vi "Analysis.FG, Data Value Items.vi"(6 "ResultID":i32, 7 "Action":T1=enum."Add Value", 8 "UL":string, 9 "LL":string, 10 "Value":string, 11 "Name":string) -> (0 "error out":errorcluster, 1 "2DVals Out":string[][](array[string]), 2 "Name/1DVals Out":string[](array[string]), 3 "Limits":variant, 4 "1DVals Num":dbl[](array[numeric]))   [LabVIEW 2024]
uses:
  Analysis.Data Value Items Action.ctl
  Analysis.Measurement Limit Info.ctl
  <vilib>/KATE/Files/File Utils.lvlib
  <vilib>/KATE/Strings/String Utils.lvlib
panel:
  # "Init\n  Clear Data\n\nAdd Value:\n  Inputs:\n    ResultID\n    Name\n    Val\n    LL\n    UL\n  Outputs:\n    None\n\nGet Meas Num Values \n  Used for Graphs\n  Inputs:\n    Name\n  Outputs:\n    1D Num Values\n       Indices align with TestResultID\n\nGet Meas Num Values Only \n  Used for Stats\n  Inputs:\n    Name\n  Outputs:\n    1D Num Values\n       Array of numeric data only\n\nDump All:\n   Outputs:\n     Var Limits\n     1D Names\n     2D Values"
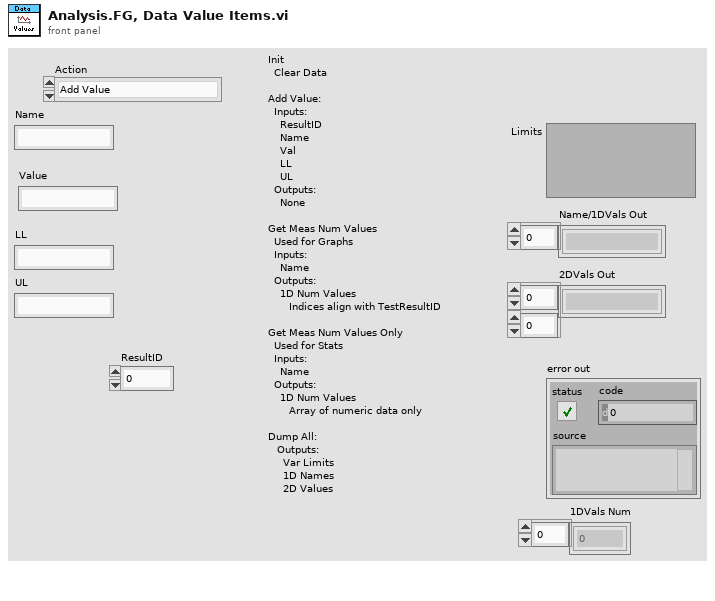
[diagram p1: front panel]
types:
  T1 = typedef "Analysis.Data Value Items Action.ctl" = enum16{"Init", "Add Value", "Get MeasVals", "Get Lists", "Get RsltVals", "Dump All", "Dump Vals to File", "Get Rslt Meas Val", "Dump Lists to File", "Load Values from File", "Load Lists From File", "Get MeasVals Num Only", "TrimDataTable"}
  T2 = typedef "Analysis.Measurement Limit Info.ctl" = cluster{"Name":string, "Numeric":bool, "LL":dbl, "LL_En":bool, "UL":dbl, "UL_En":bool, "Units":string}
  T3 = enum16{"open", "replace", "create", "open or create", "replace or create", "replace or create with confirmation"}
  T4 = cluster{"Names":string[], "MeasDims_Out":variant}
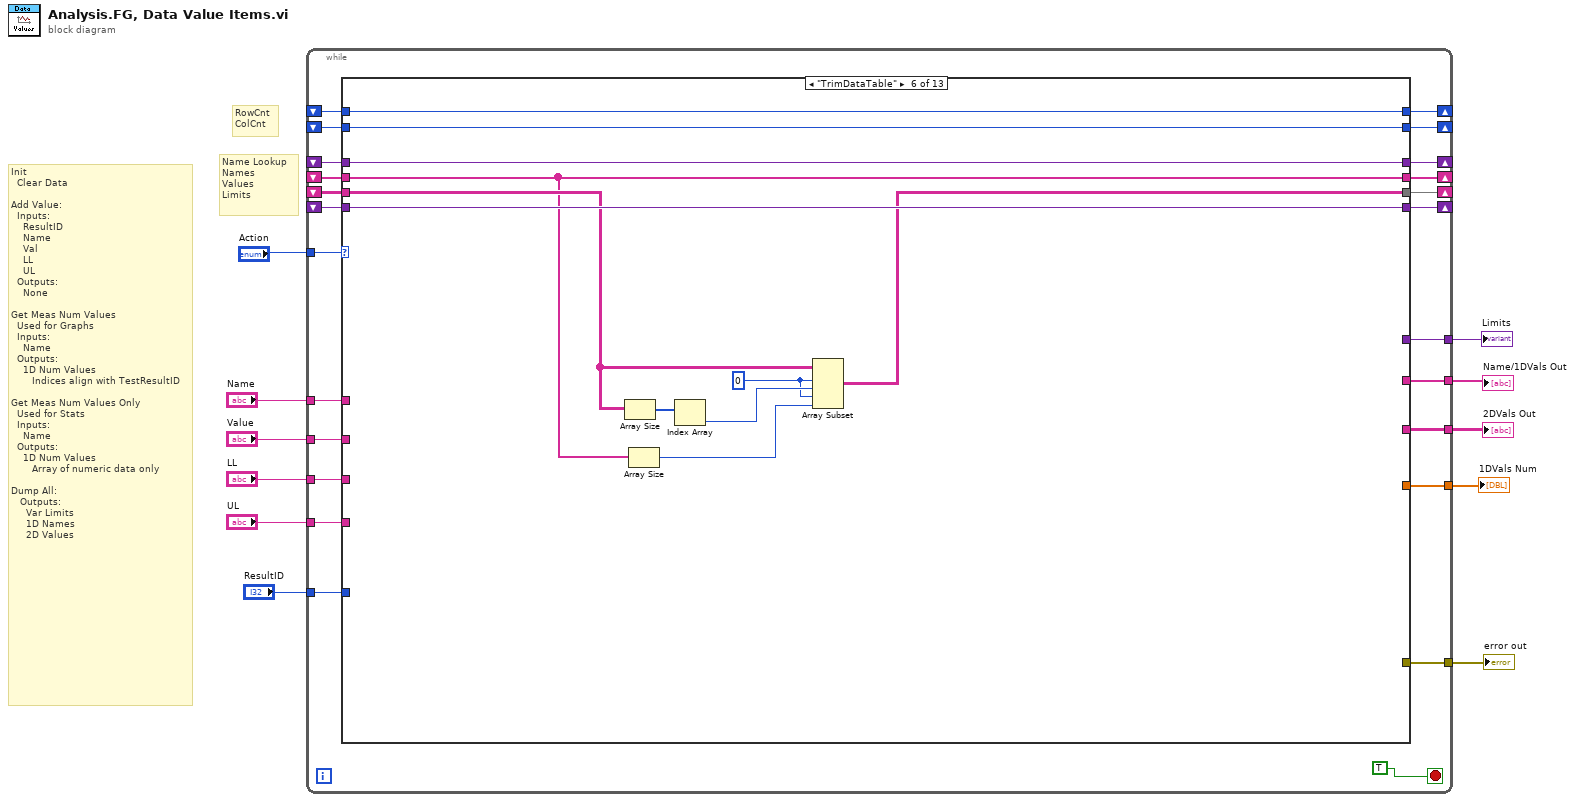
[diagram p0: block diagram]
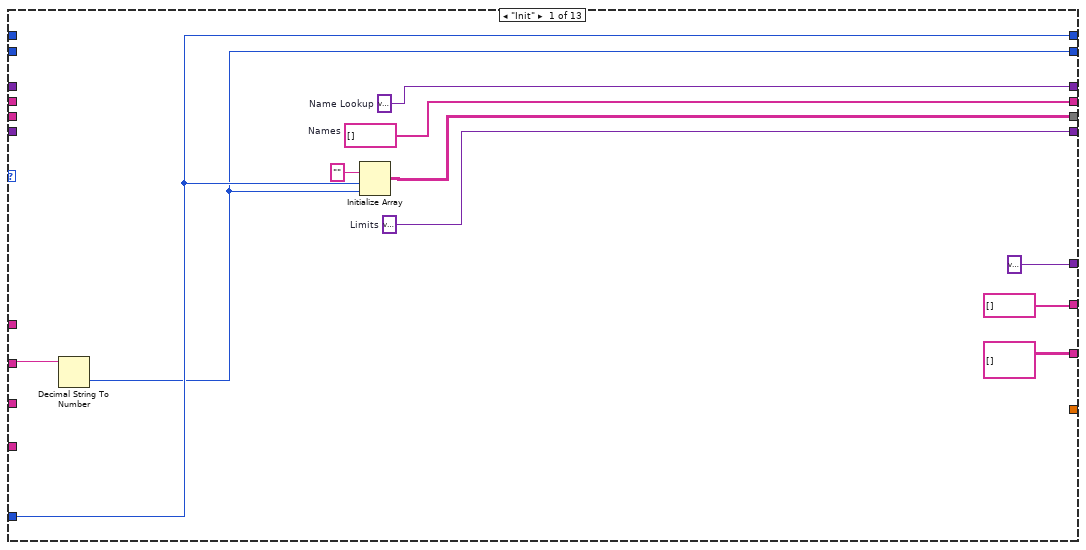
[diagram p2: hidden frame]
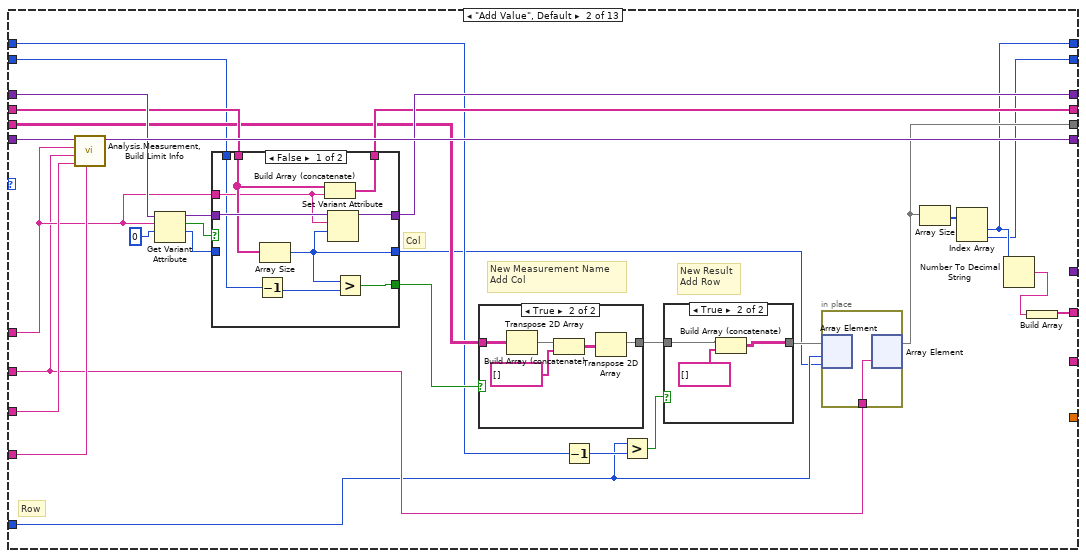
[diagram p3: hidden frame]
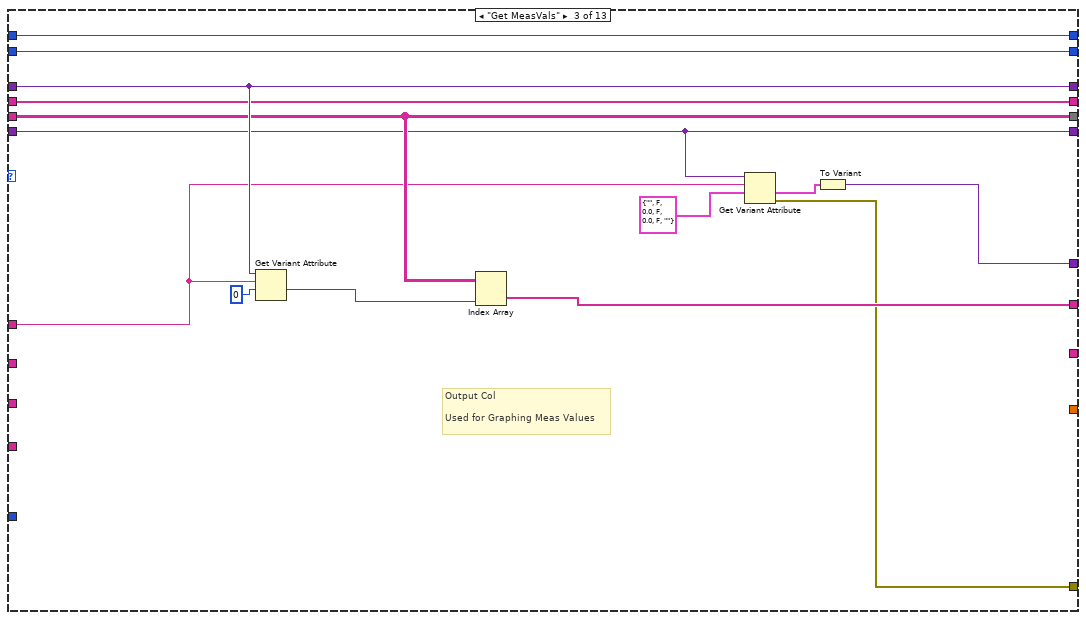
[diagram p7: hidden frame]
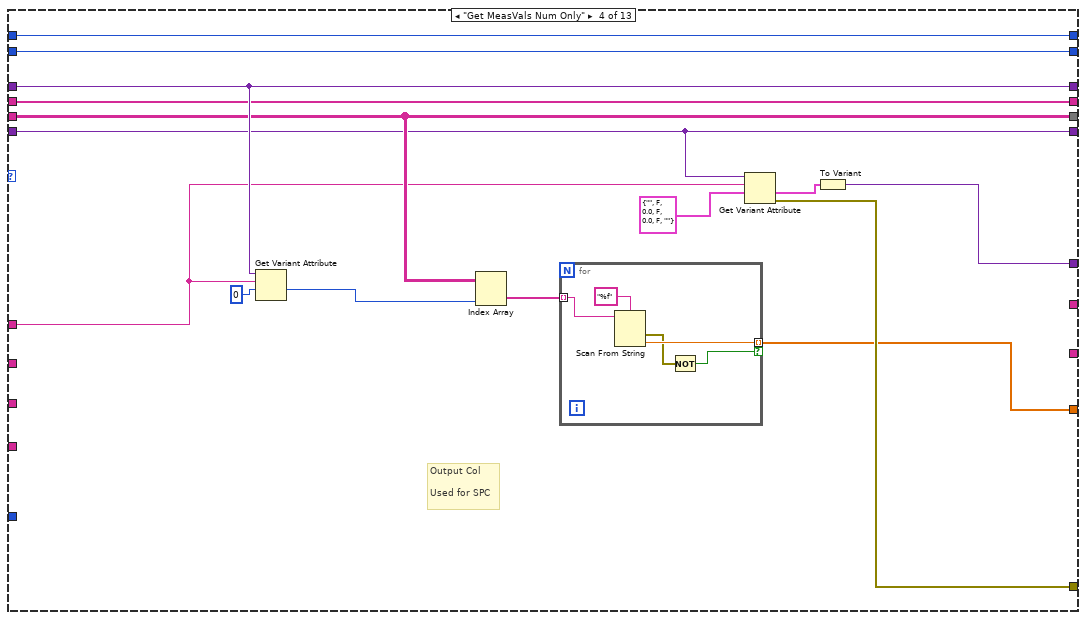
[diagram p8: hidden frame]
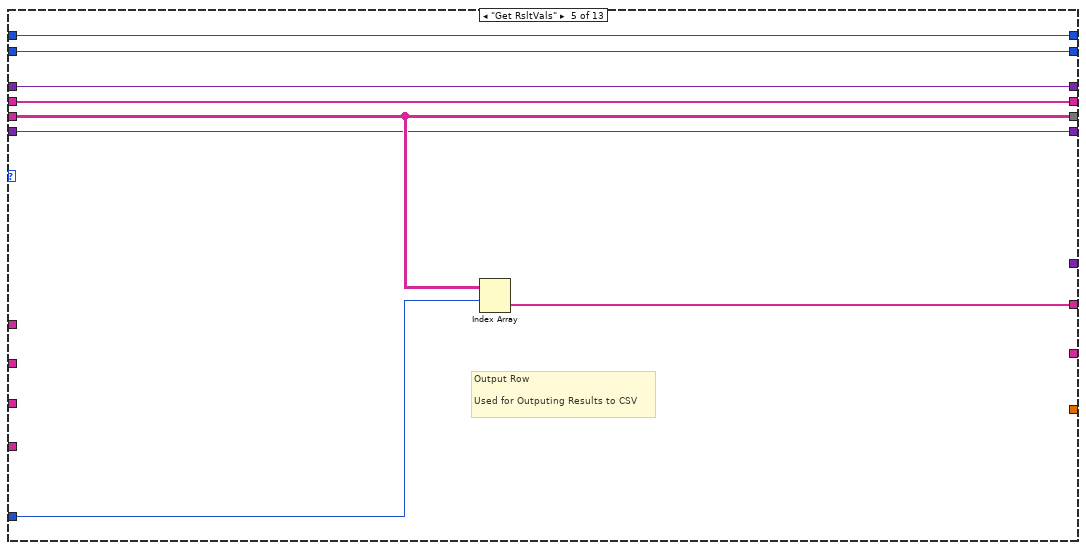
[diagram p9: hidden frame]
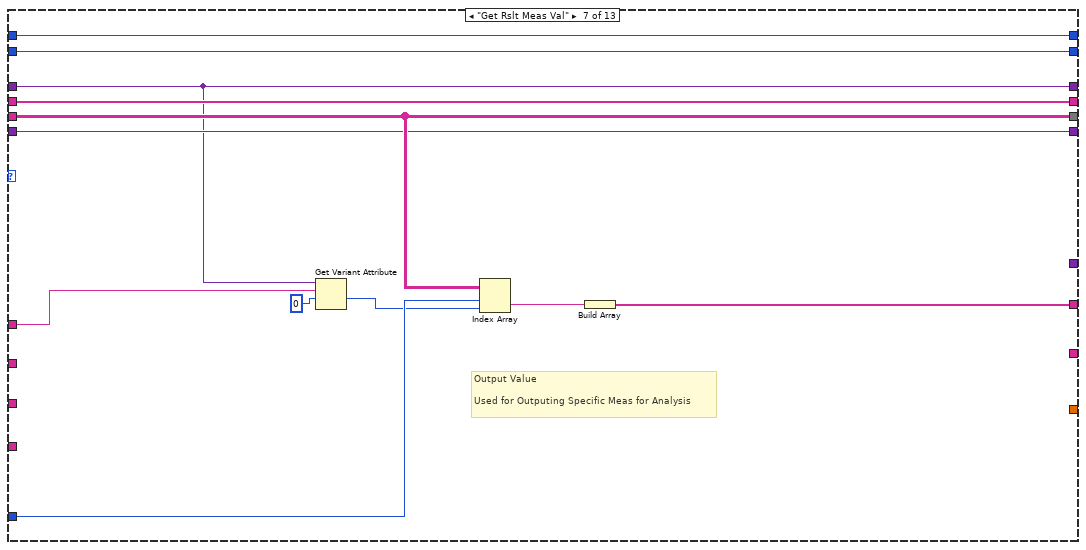
[diagram p10: hidden frame]
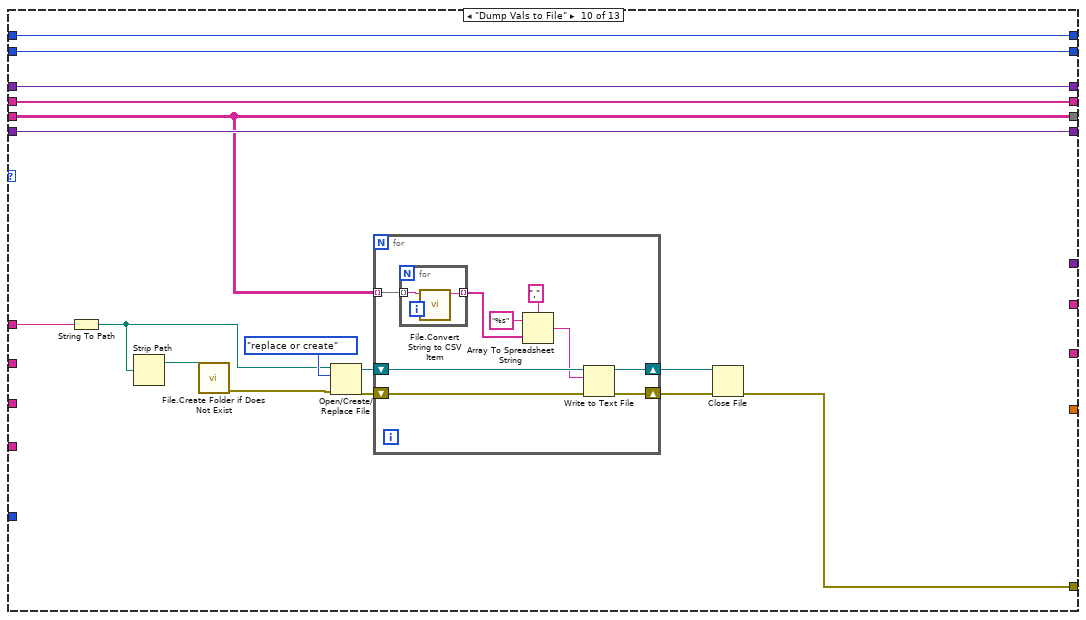
[diagram p13: hidden frame]
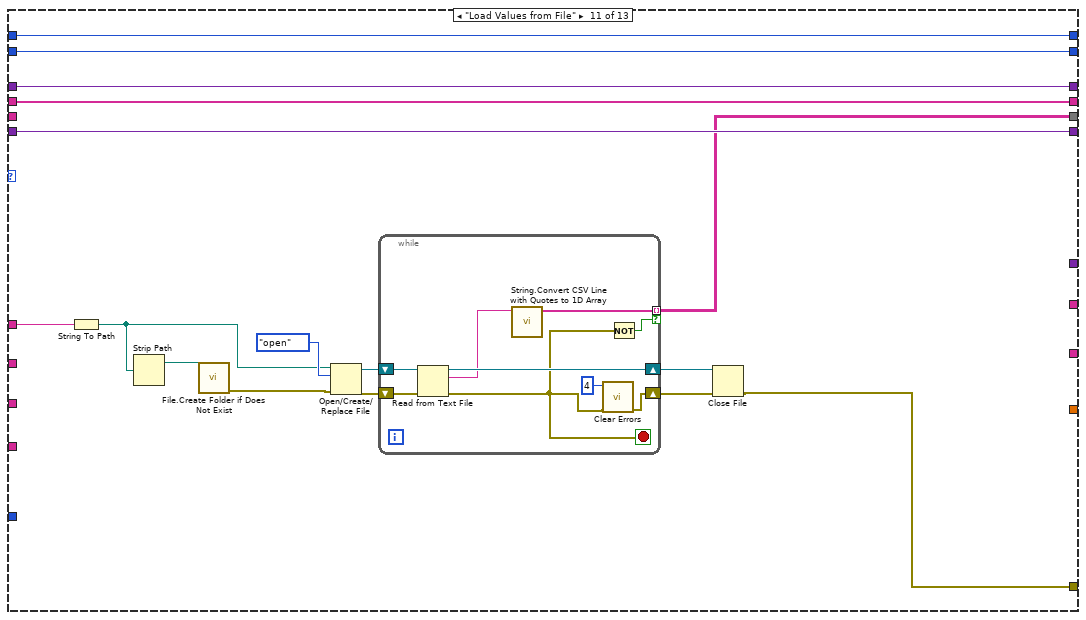
[diagram p14: hidden frame]
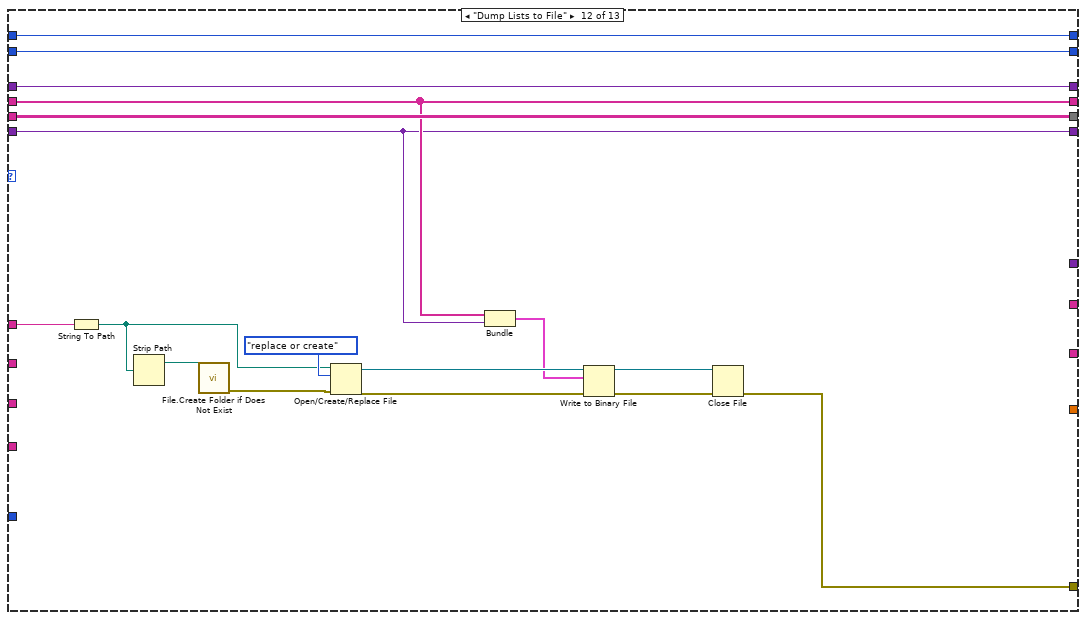
[diagram p15: hidden frame]
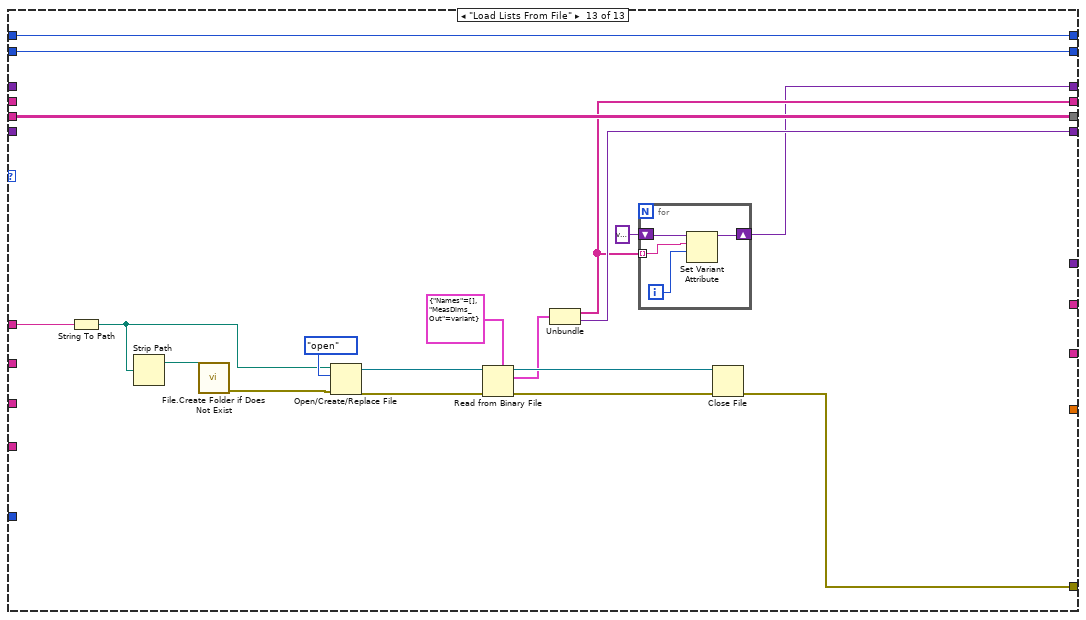
[diagram p16: hidden frame]
diagram:
  # "RowCnt\nColCnt"
  # "Init\n  Clear Data\n\nAdd Value:\n  Inputs:\n    ResultID\n    Name\n    Val\n    LL\n    UL\n  Outputs:\n    None\n\nGet Meas Num Values \n  Used for Graphs\n  Inputs:\n    Name\n  Outputs:\n    1D Num Values\n       Indices align with TestResultID\n\nGet Meas Num Values Only \n  Used for Stats\n  Inputs:\n    Name\n  Outputs:\n    1D Num Values\n       Array of numeric data only\n\nDump All:\n   Outputs:\n     Var Limits\n     1D Names\n     2D Values"
  # "Name Lookup\nNames\nValues\nLimits"
  n1 = while {
    tunnel: "Action" -> [w35]
    shift-right: [w29] -> _
    shift-left: _ -> [w34]
    shift-right: [w28] -> _
    shift-left: _ -> [w33]
    shift-right: [w27] -> _
    shift-left: _ -> [w32]
    shift-right: [w30] -> _
    shift-left: _ -> [w31]
    tunnel: "ResultID" -> [w26]
    tunnel: "Name" -> [w25]
    tunnel: "Value" -> [w24]
    tunnel: "LL" -> [w23]
    tunnel: "UL" -> [w22]
    tunnel: [w21] -> w5
    tunnel: [w20] -> w4
    tunnel: [w19] -> w3
    tunnel: [w17] -> w2
    tunnel: [w16] -> w1
    shift-right: [w15] -> _
    shift-left: _ -> [w13]
    shift-right: [w14] -> _
    shift-left: _ -> [w12]
    stop <- TRUE stop-if-true
    n2 = case shown="\"TrimDataTable\"" w35 {
      tunnel: w34 -> [_ w76 w107 w123 w139 w151 w163 w167 w175 w191 w218 w233 _]
      tunnel: [w37 w49 w111 w126 w140 w142 w164 w170 w173 w180 w207 w235 w255] -> w28
      tunnel: [w46 w66 w109 w124 w138 w144 w162 w168 w174 w190 w217 w234 w250] -> w27
      tunnel: w33 -> [_ w60 w111 w126 w140 w148 w164 w170 w173 w180 _ w235 w255]
      tunnel: w32 -> [_ w67 w109 w124 w138 w144 w162 w168 w174 w190 w217 w234 _]
      tunnel: w31 -> [_ w70 w112 w127 w141 w152 w159 w169 w176 w192 w219 w245 _]
      tunnel: [w45 w69 w112 w127 w141 w152 w159 w169 w176 w192 w219 w245 w248] -> w30
      tunnel: [w44 w73 w107 w123 w139 w151 w163 w167 w175 w191 w218 w233 w252] -> w29
      tunnel: w26 -> [w40 w51 _ _ w137 _ w161 _ _ _ _ _ _]
      tunnel: w25 -> [_ w68 w105 w121 _ _ w158 _ _ w189 w216 w244 w264]
      tunnel: w24 -> [w36 w52 _ _ _ _ _ _ _ _ _ _ _]
      tunnel: w23 -> [_ w75 _ _ _ _ _ _ _ _ _ _ _]
      tunnel: w22 -> [_ w74 _ _ _ _ _ _ _ _ _ _ _]
      tunnel: [variant ("Var Out") _ w102 w118 _ _ _ w167 w175 _ _ _ _] -> w21
      tunnel: [string[] [] ("1D Str Out") w57 w108 _ w136 _ w155 w168 w174 _ _ _ _] -> w20
      tunnel: [string[][] [] ("2D Str Out") _ _ _ _ _ _ _ w173 _ _ _ _] -> w19
      tunnel: [_ _ w104 w120 _ _ _ _ _ w179 w206 w231 w251] -> w17
      tunnel: [_ _ _ w116 _ _ _ _ _ _ _ _ _] -> w16
      tunnel: [w40 w48 w101 w115 w135 w150 w154 w166 w172 w178 w205 w230 w247] -> w15
      tunnel: [w39 w47 w100 w114 w134 w149 w153 w165 w171 w177 w204 w229 w246] -> w14
      tunnel: w13 -> [_ w55 w101 w115 w135 w150 w154 w166 w172 w178 w205 w230 w247]
      tunnel: w12 -> [_ w54 w100 w114 w134 w149 w153 w165 w171 w177 w204 w229 w246]
      frame "Init" {
        w45 = variant  # Name Lookup
        w44 = variant  # Limits
        w46 = string[] []  # Names
        n3 = Decimal String To Number(string=w36) -> (number=w39:i32)  [unwired: 2 in, 1 out]
        n4 = Initialize Array("", w40, w39) -> (w37:string[][])
      }
      frame "Add Value", Default {
        # "New Measurement Name\nAdd Col"
        # "New Result\nAdd Row"
        # "Col"
        # "Row"
        n5 = call "Analysis.Measurement, Build Limit Info.vi"("UL"=w74, "LL"=w75, "Value"=w52, "Name"=w68, "MeasDims_In"=w76) -> ("MeasDims_Out"=w73:variant)  [unwired: 5 in, 1 out]
        n6 = Get Variant Attribute(Variant=w70, name=w68, default value (empty Variant)=0) -> (duplicate Variant=w72:variant, found=w71:bool, value=w64:i32)  [unwired: 1 in, 1 out]
        n7 = case shown="False" w71 {
          tunnel: w72 -> [w95 w99]
          tunnel: [w96 w99] -> w69
          tunnel: w68 -> [w92 _]
          tunnel: w67 -> [w94 w98]
          tunnel: [w93 w98] -> w66
          tunnel: w64 -> [_ w97]
          tunnel: [w90 w97] -> w50
          tunnel: [w88 _] -> w59
          tunnel: w54 -> [w91 _]
          frame False {
            n8 = Decrement(x=w91) -> (x-1=w89:i32)
            n9 = Array Size(array=w94) -> (size(s)=w90:i32)
            n10 = Build Array (concatenate)(w94, w92) -> (w93:string[])
            n11 = Set Variant Attribute(Variant=w95, name=w92, value=w90) -> (Variant out=w96:variant)  [unwired: 1 in, 2 out]
            n12 = Greater?(x=w90, y=w89) -> (0:w88:bool)
          }
          frame True {
            # "Do Nothing"
          }
        }
        n13 = case shown="True" w59 {
          tunnel: w60 -> [w82 w86]
          tunnel: [w82 w83] -> w63
          frame False {
          }
          frame True {
            n14 = Transpose 2D Array(2D array=w86) -> (transposed array=w85:string[][])
            n15 = Build Array (concatenate)(w85, string[] []) -> (w84:string[][])
            n16 = Transpose 2D Array(2D array=w84) -> (transposed array=w83:string[][])
          }
        }
        n17 = Decrement(x=w55) -> (x-1=w61:i32)
        n18 = Greater?(x=w51, y=w61) -> (0:w62:bool)
        n19 = case shown="True" w62 {
          tunnel: w63 -> [w78 w81]
          tunnel: [w78 w79] -> w53
          frame False {
          }
          frame True {
            n20 = Build Array (concatenate)(w81, string[] []) -> (w79:string[][])
          }
        }
        n21 = in-place {
          in-place-border: w52 -> [w77]
          n22 = in-place-array #1(w53, w51, w50) -> ()  [unwired: 1 out]
          n23 = in-place-array #1(w77) -> (w49:string[][])  [unwired: 2 out]
        }
        n24 = Array Size(array=w49) -> (size(s)=w58:i32[])
        n25 = Index Array(array=w58) -> (element #1=w48:i32, element #2=w47:i32)  [unwired: 2 in]
        n26 = Number To Decimal String(number=w48) -> (decimal integer string=w56:string)  [unwired: 1 in]
        n27 = Build Array(w56) -> (w57:string[])
      }
      frame "Get MeasVals" {
        # "Output Col\n\nUsed for Graphing Meas Values"
        n28 = Get Variant Attribute(Variant=w112, name=w105, default value (empty Variant)=0) -> (value=w110:i32)  [unwired: 1 in, 3 out]
        n29 = Index Array(array=w111, index (col)=w110) -> (element=w108:string[])  [unwired: 1 in]
        n30 = Get Variant Attribute(Variant=w107, name=w105, default value (empty Variant)=T2 {"Name"="", "Numeric"=FALSE, "LL"=0.0, "LL_En"=FALSE, "UL"=0.0, "UL_En"=FALSE, "Units"=""} ("Measurement Dimension")) -> (value=w103:T2, error out=w104:errorcluster)  [unwired: 1 in, 2 out]
        n31 = To Variant(anything=w103) -> (Variant=w102:variant)
      }
      frame "Get MeasVals Num Only" {
        # "Output Col\n\nUsed for SPC"
        n32 = Get Variant Attribute(Variant=w127, name=w121, default value (empty Variant)=0) -> (value=w125:i32)  [unwired: 1 in, 3 out]
        n33 = Index Array(array=w126, index (col)=w125) -> (element=w117:string[])  [unwired: 1 in]
        n34 = for {
          tunnel: w117 -> [w132] mode=indexing
          tunnel: [w131] -> w116 mode=indexing if=w129
          n35 = Scan From String(format string="%f", input string=w132) -> (error out=w130:errorcluster, output 1=w131:dbl)  [unwired: 3 in, 2 out]
          n36 = Not(x=w130) -> (.not. x?=w129:bool)
        }
        n37 = Get Variant Attribute(Variant=w123, name=w121, default value (empty Variant)=T2 {"Name"="", "Numeric"=FALSE, "LL"=0.0, "LL_En"=FALSE, "UL"=0.0, "UL_En"=FALSE, "Units"=""} ("Measurement Dimension")) -> (value=w119:T2, error out=w120:errorcluster)  [unwired: 1 in, 2 out]
        n38 = To Variant(anything=w119) -> (Variant=w118:variant)
      }
      frame "Get RsltVals" {
        # "Output Row\n\nUsed for Outputing Results to CSV"
        n39 = Index Array(array=w140, index (row)=w137) -> (element=w136:string[])  [unwired: 1 in]
      }
      frame "TrimDataTable" {
        w145 = 0 ("index")
        n40 = Array Size(array=w148) -> (size(s)=w147:i32[])
        n41 = Array Size(array=w144) -> (size(s)=w143:i32)
        n42 = Index Array(array=w147) -> (element=w146:i32)  [unwired: 1 in]
        n43 = Array Subset(array=w148, index (row)=w145, length (row)=w146, index (col)=w145, length (col)=w143) -> (w142:string[][])
      }
      frame "Get Rslt Meas Val" {
        # "Output Value\n\nUsed for Outputing Specific Meas for Analysis"
        n44 = Get Variant Attribute(Variant=w159, name=w158, default value (empty Variant)=0) -> (value=w157:i32)  [unwired: 1 in, 3 out]
        n45 = Index Array(array=w164, index (row)=w161, index (col)=w157) -> (element=w156:string)
        n46 = Build Array(w156) -> (w155:string[])
      }
      frame "Get Lists" {
      }
      frame "Dump All" {
      }
      frame "Dump Vals to File" {
        n47 = String To Path(string=w189) -> (path=w182:path)
        n48 = Strip Path(path=w182) -> (stripped path=w188:path)  [unwired: 1 out]
        n49 = call <vilib>:"File.Create Folder if Does Not Exist.vi"("Path"=w188) -> ("error out"=w181:errorcluster)  [unwired: 8 in, 2 out]
        n50 = Open/Create/Replace File(file path (use dialog)=w182, error in=w181, operation (0:open)=T3."replace or create") -> (refnum out=w185:refnum<file>, error out=w184:errorcluster)  [unwired: 3 in, 1 out]
        n51 = for {
          shift-right: [w200] -> w187
          shift-left: w185 -> [w198]
          shift-right: [w199] -> w186
          shift-left: w184 -> [w196]
          tunnel: w180 -> [w195] mode=indexing
          n52 = for {
            tunnel: w195 -> [w202] mode=indexing
            tunnel: [w203] -> w194 mode=indexing
            n53 = call <vilib>:"File.Convert String to CSV Item.vi"("String"=w202) -> ("String Out"=w203:string)  [unwired: 10 in]
          }
          n54 = Array To Spreadsheet String(delimiter (Tab)=",", array=w194, 3:"%s" ("format string")) -> (spreadsheet string=w197:string)
          n55 = Write to Text File(file (use dialog)=w198, text=w197, error in=w196) -> (refnum out=w200:refnum<file>, error out=w199:errorcluster)  [unwired: 1 in, 1 out]
        }
        n56 = Close File(refnum=w187, error in=w186) -> (error out=w179:errorcluster)  [unwired: 1 out]
      }
      frame "Load Values from File" {
        n57 = String To Path(string=w216) -> (path=w209:path)
        n58 = Strip Path(path=w209) -> (stripped path=w215:path)  [unwired: 1 out]
        n59 = call <vilib>:"File.Create Folder if Does Not Exist.vi"("Path"=w215) -> ("error out"=w208:errorcluster)  [unwired: 8 in, 2 out]
        n60 = Open/Create/Replace File(file path (use dialog)=w209, error in=w208, operation (0:open)=T3."open") -> (refnum out=w212:refnum<file>, error out=w211:errorcluster)  [unwired: 3 in, 1 out]
        n61 = while {
          shift-right: [w228] -> w214
          shift-left: w212 -> [w227]
          shift-right: [w220] -> w213
          shift-left: w211 -> [w226]
          tunnel: [w224] -> w207 mode=indexing if=w223
          stop <- w221 stop-if-true
          n62 = Read from Text File(file (use dialog)=w227, error in=w226) -> (refnum out=w228:refnum<file>, text=w225:string, error out=w221:errorcluster)  [unwired: 2 in, 1 out]
          n63 = call <vilib>:"String.Convert CSV Line with Quotes to 1D Array.vi"("CSV String"=w225) -> ("Array"=w224:string[])  [unwired: 9 in, 1 out]
          n64 = call <vilib>:"Clear Errors.vi"("error in (no error)"=w221, "specific error code to clear (0: all)"=4) -> ("error out"=w220:errorcluster)  [unwired: 4 in, 1 out]
          n65 = Not(x=w221) -> (.not. x?=w223:bool)
        }
        n66 = Close File(refnum=w214, error in=w213) -> (error out=w206:errorcluster)  [unwired: 1 out]
      }
      frame "Dump Lists to File" {
        n67 = String To Path(string=w244) -> (path=w237:path)
        n68 = Strip Path(path=w237) -> (stripped path=w243:path)  [unwired: 1 out]
        n69 = call <vilib>:"File.Create Folder if Does Not Exist.vi"("Path"=w243) -> ("error out"=w236:errorcluster)  [unwired: 8 in, 2 out]
        n70 = Open/Create/Replace File(file path (use dialog)=w237, error in=w236, operation (0:open)=T3."replace or create") -> (refnum out=w240:refnum<file>, error out=w239:errorcluster)  [unwired: 3 in, 1 out]
        n71 = Bundle("Names"=w234, "MeasDims_Out"=w233) -> (w232:T4)  [unwired: 1 in]
        n72 = Write to Binary File(file (use dialog)=w240, data=w232, error in=w239) -> (refnum out=w242:refnum<file>, error out=w241:errorcluster)  [unwired: 3 in, 1 out]
        n73 = Close File(refnum=w242, error in=w241) -> (error out=w231:errorcluster)  [unwired: 1 out]
      }
      frame "Load Lists From File" {
        n74 = String To Path(string=w264) -> (path=w257:path)
        n75 = Strip Path(path=w257) -> (stripped path=w263:path)  [unwired: 1 out]
        n76 = call <vilib>:"File.Create Folder if Does Not Exist.vi"("Path"=w263) -> ("error out"=w256:errorcluster)  [unwired: 8 in, 2 out]
        n77 = Open/Create/Replace File(file path (use dialog)=w257, error in=w256, operation (0:open)=T3."open") -> (refnum out=w260:refnum<file>, error out=w259:errorcluster)  [unwired: 3 in, 1 out]
        n78 = Read from Binary File(5:T4 {"Names"=[], "MeasDims_Out"=variant} ("output cluster"), 8:w259, 11:w260) -> (0:w261:errorcluster, 2:w254:T4, 3:w262:refnum<file>)  [unwired: 3 in, 1 out]
        n79 = Unbundle(w254) -> ("Names"=w250:string[], "MeasDims_Out"=w252:variant)
        n80 = for {
          tunnel: w250 -> [w265] mode=indexing
          shift-right: [w267] -> w248
          shift-left: variant -> [w268]
          i -> [w266]
          n81 = Set Variant Attribute(Variant=w268, name=w265, value=w266) -> (Variant out=w267:variant)  [unwired: 1 in, 2 out]
        }
        n82 = Close File(refnum=w262, error in=w261) -> (error out=w251:errorcluster)  [unwired: 1 out]
      }
    }
  }
  "Name/1DVals Out" <- w4
  "2DVals Out" <- w3
  "Limits" <- w5
  "error out" <- w2
  "1DVals Num" <- w1
